vi "QVA_GetAttributesToModify.vi"(0 "QueueIn":refnum<queue>, 2 "Timeout":i32=-1, 5 "ErrorIn":errorcluster) -> (14 "QueueOut":refnum<queue>, 16 "Timeout":bool, 17 "VariantData":variant, 19 "ErrorOut":errorcluster)   [LabVIEW 2016]
doc: "Holt sich das Queue Element zur Bearbeitung. Danach muss zwingend SetAttributesWhenModified.vi aufgerufen werden, damit die Variable wieder freidegeben wird.\n\nsige / 3.12.13"
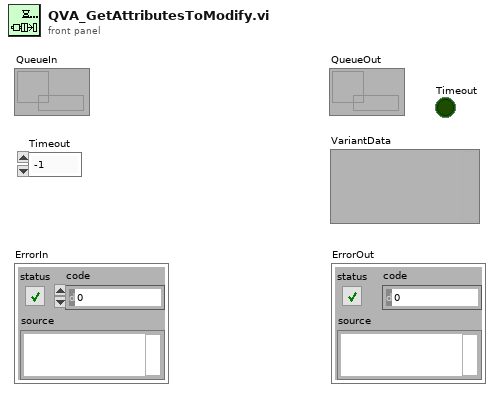
[diagram p1: front panel]
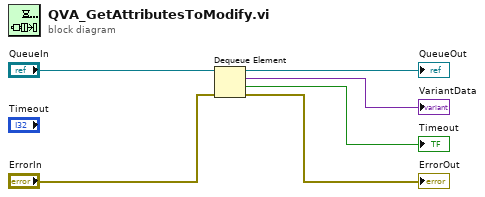
[diagram p0: block diagram]
diagram:
  n1 = Dequeue Element(queue="QueueIn", error in (no error)="ErrorIn") -> (queue out=→"QueueOut":refnum<queue>, element=→"VariantData":variant, timed out?=→"Timeout":bool, error out=→"ErrorOut":errorcluster)  [unwired: 1 in]
